vi "실습 8-2 글로벌 변수.vi"() -> ()   [LabVIEW 2014]
panel:
  in  "정지":bool
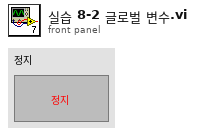
[diagram p1: front panel]
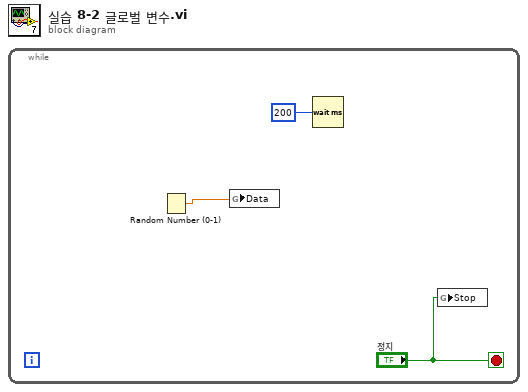
[diagram p0: block diagram]
diagram:
  n1 = while {
    stop <- "정지" stop-if-true
    n2 = Random Number (0-1)() -> (number: 0 to 1=w3:dbl)
    n3 = global write "my글로벌.vi" "Data"(w3) -> ()
    n4 = Wait (ms)(milliseconds to wait=u32 200 ("대기 시간(ms)")) -> ()  [unwired: 1 out]
    n5 = global write "my글로벌.vi" "Stop"("정지") -> ()
  }
